vi "get_all_logic_statements.vi"(8 "error in (no error)":errorcluster, 11 "VISA resource name":refnum<visa-resource-name>) -> (0 "error out":errorcluster, 2 "All logic statements":string[](array[string]), 3 "VISA resource name out":refnum<visa-resource-name>)   [LabVIEW 2018]
doc: "Update all logic statements."
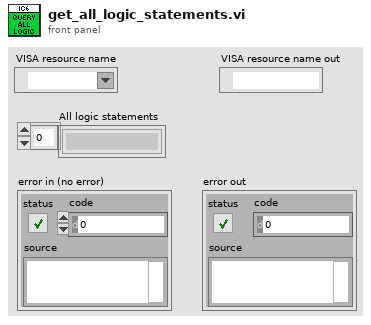
[diagram p1: front panel]
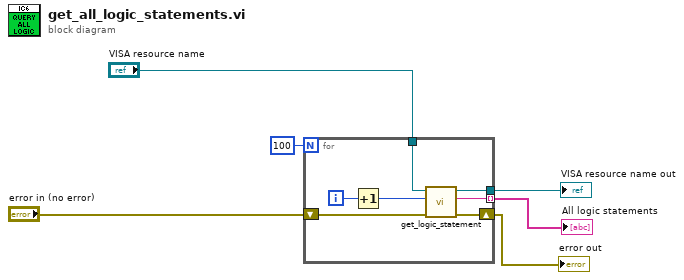
[diagram p0: block diagram]
diagram:
  n1 = for {
    N: 100 -> [_]
    tunnel: "VISA resource name" -> [w11]
    shift-right: [w9] -> w6
    shift-left: "error in (no error)" -> [w10]
    tunnel: [w8] -> w4
    tunnel: [w7] -> w1 mode=indexing
    i -> [w13]
    n2 = Increment(x=w13) -> (x+1=w12:i32)
    n3 = call "get_logic_statement.vi"("error in (no error)"=w10, "Statement number"=w12, "VISA resource name"=w11) -> ("error out"=w9:errorcluster, "Logic statement"=w7:string, "VISA resource name out"=w8:refnum<visa-resource-name>)  [unwired: 6 in]
  }
  "error out" <- w6
  "All logic statements" <- w1
  "VISA resource name out" <- w4
